vi "niFpga wdp fft apply twid factors.vi"(6 "enable":bool, 8 "data index 1":fxp<+,9,9>, 9 "data index 0":fxp<+,9,9>, 10 "data in 1":T1(array[cluster])=[{"data re"=0.0, "data im"=0.0}, {"data re"=0.0, "data im"=0.0}, {"data re"=0.0, "data im"=0.0}, {"data re"=0.0, "data im"=0.0}, {"data re"=0.0, "data im"=0.0}, {"data re"=0.0, "data im"=0.0}, {"data re"=0.0, "data im"=0.0}, {"data re"=0.0, "data im"=0.0}], 11 "data in 0":T1(array[cluster])=[{"data re"=0.0, "data im"=0.0}, {"data re"=0.0, "data im"=0.0}, {"data re"=0.0, "data im"=0.0}, {"data re"=0.0, "data im"=0.0}, {"data re"=0.0, "data im"=0.0}, {"data re"=0.0, "data im"=0.0}, {"data re"=0.0, "data im"=0.0}, {"data re"=0.0, "data im"=0.0}]) -> (2 "data out 1":T1(array[cluster]), 3 "data out 0":T1(array[cluster]))   [LabVIEW 2017]
types:
  T1 = cluster{"data re":fxp<+/-,8,1>, "data im":fxp<+/-,8,1>}[]
  T2 = cluster{"data re":fxp<+/-,8,1>, "data im":fxp<+/-,8,1>}
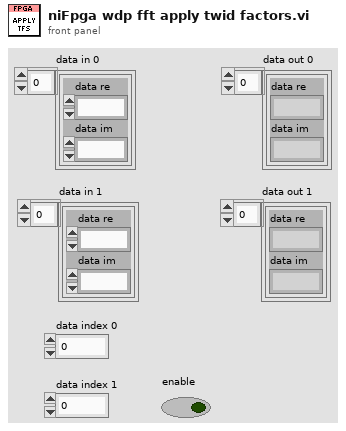
[diagram p1: front panel]
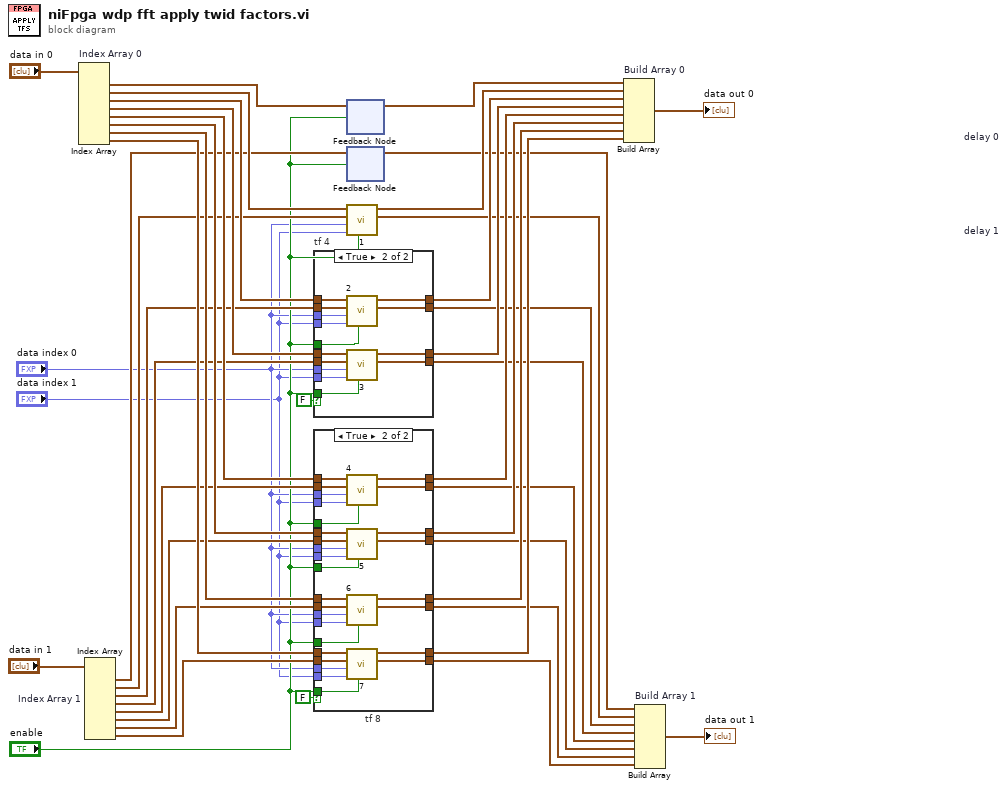
[diagram p0: block diagram]
diagram:
  n1 = Index Array "Index Array 0"(array="data in 0") -> (element #1=w39:T2, element #2=w36:T2, element #3=w35:T2, element #4=w34:T2, element #5=w33:T2, element #6=w32:T2, element #7=w31:T2, element #8=w30:T2)  [unwired: 8 in]
  n2 = Index Array "Index Array 1"(array="data in 1") -> (element #1=w29:T2, element #2=w28:T2, element #3=w27:T2, element #4=w26:T2, element #5=w25:T2, element #6=w24:T2, element #7=w23:T2, element #8=w22:T2)  [unwired: 8 in]
  n3 = case "tf 4" shown="True" FALSE {
    tunnel: w35 -> [_ w55]
    tunnel: w34 -> [_ w54]
    tunnel: w27 -> [_ w53]
    tunnel: w26 -> [_ w52]
    tunnel: "data index 0" -> [_ w51]
    tunnel: "data index 0" -> [_ w50]
    tunnel: "data index 1" -> [_ w49]
    tunnel: "data index 1" -> [_ w48]
    tunnel: [_ w47] -> w19
    tunnel: [_ w46] -> w18
    tunnel: [_ w45] -> w11
    tunnel: [_ w44] -> w10
    tunnel: "enable" -> [_ w43]
    tunnel: "enable" -> [_ w42]
    frame False {
    }
    frame True {
      n4 = call "2"("enable"=w42, "data index 1"=w49, "data index 0"=w51, "data in 1"=w53, "data in 0"=w55) -> ("data out 1"=w45:T2, "data out 0"=w47:T2)  [unwired: 5 in]
      n5 = call "3"("enable"=w43, "data index 1"=w48, "data index 0"=w50, "data in 1"=w52, "data in 0"=w54) -> ("data out 1"=w44:T2, "data out 0"=w46:T2)  [unwired: 5 in]
    }
  }
  n6 = case "tf 8" shown="True" FALSE {
    tunnel: w33 -> [_ w83]
    tunnel: w32 -> [_ w82]
    tunnel: w31 -> [_ w81]
    tunnel: w30 -> [_ w80]
    tunnel: w25 -> [_ w79]
    tunnel: w24 -> [_ w78]
    tunnel: w23 -> [_ w77]
    tunnel: w22 -> [_ w76]
    tunnel: "data index 0" -> [_ w75]
    tunnel: "data index 0" -> [_ w74]
    tunnel: "data index 0" -> [_ w73]
    tunnel: "data index 0" -> [_ w72]
    tunnel: "data index 1" -> [_ w71]
    tunnel: "data index 1" -> [_ w70]
    tunnel: "data index 1" -> [_ w69]
    tunnel: "data index 1" -> [_ w68]
    tunnel: [_ w67] -> w17
    tunnel: [_ w66] -> w16
    tunnel: [_ w65] -> w15
    tunnel: [_ w64] -> w14
    tunnel: [_ w63] -> w9
    tunnel: [_ w62] -> w8
    tunnel: [_ w61] -> w7
    tunnel: [_ w60] -> w6
    tunnel: "enable" -> [_ w59]
    tunnel: "enable" -> [_ w58]
    tunnel: "enable" -> [_ w57]
    tunnel: "enable" -> [_ w56]
    frame False {
    }
    frame True {
      n7 = call "4"("enable"=w59, "data index 1"=w71, "data index 0"=w75, "data in 1"=w79, "data in 0"=w83) -> ("data out 1"=w63:T2, "data out 0"=w67:T2)  [unwired: 5 in]
      n8 = call "5"("enable"=w58, "data index 1"=w70, "data index 0"=w74, "data in 1"=w78, "data in 0"=w82) -> ("data out 1"=w62:T2, "data out 0"=w66:T2)  [unwired: 5 in]
      n9 = call "6"("enable"=w57, "data index 1"=w69, "data index 0"=w73, "data in 1"=w77, "data in 0"=w81) -> ("data out 1"=w61:T2, "data out 0"=w65:T2)  [unwired: 5 in]
      n10 = call "7"("enable"=w56, "data index 1"=w68, "data index 0"=w72, "data in 1"=w76, "data in 0"=w80) -> ("data out 1"=w60:T2, "data out 0"=w64:T2)  [unwired: 5 in]
    }
  }
  n11 = feedback #1 "delay 0"() -> (w21:T2)  [unwired: 1 in]
  n12 = feedback-in #1(w39, "enable") -> ()
  n13 = feedback #2 "delay 1"() -> (w13:T2)  [unwired: 1 in]
  n14 = feedback-in #2(w29, "enable") -> ()
  n15 = call "1"("enable"="enable", "data index 1"="data index 1", "data index 0"="data index 0", "data in 1"=w28, "data in 0"=w36) -> ("data out 1"=w12:T2, "data out 0"=w20:T2)  [unwired: 5 in]
  n16 = Build Array "Build Array 0"(w21, w20, w19, w18, w17, w16, w15, w14) -> (→"data out 0":T1)
  n17 = Build Array "Build Array 1"(w13, w12, w11, w10, w9, w8, w7, w6) -> (→"data out 1":T1)
